vi "stop.vi"(8 "error in (no error)":errorcluster, 10 "stop?":bool, 11 "BECHWCBasic in":refnum<class "BECHWCBasic.lvclass">) -> (0 "error out":errorcluster, 2 "stopped":bool, 3 "BECHWCBasic out":refnum<class "BECHWCBasic.lvclass">)   [LabVIEW 2011, in "Hardware.lvlib" / "HWControllers.lvlib" / "BECHWCBasic.lvclass"]
doc: "Stop current run if input is true, otherwise ask hardware if its finished."
uses:
  BECHWCBasic.lvclass
  BECHWCBasic.lvclass/BECHWCBasic.ctl
  Channels/Digital/DigitalOutput.lvclass
  Channels/VoltOutput/AnalogOutput.lvclass
  IntegrationManagement/CameraManager.lvclass
  HWController.lvclass
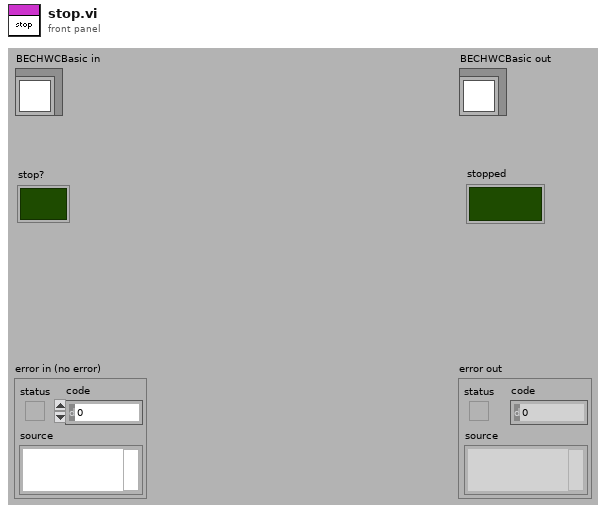
[diagram p1: front panel]
types:
  T1 = enum16{"Ready", "Compiling", "Configured", "Running", "Stopping", "Unresolved Error"}
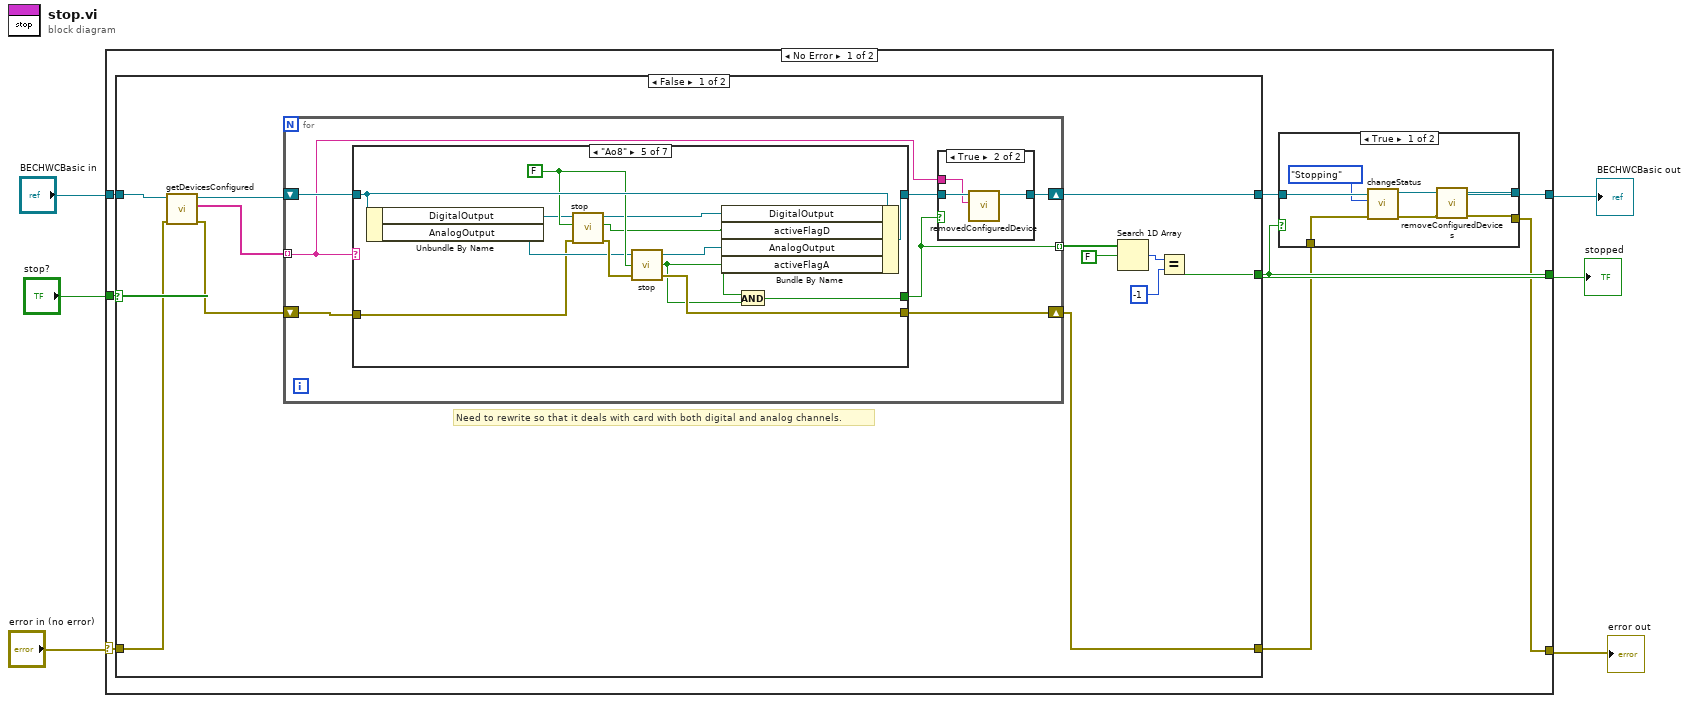
[diagram p0: block diagram]
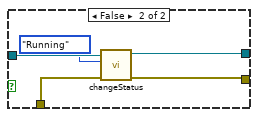
[diagram p2: hidden frame]
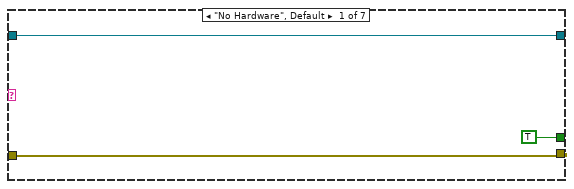
[diagram p4: hidden frame]
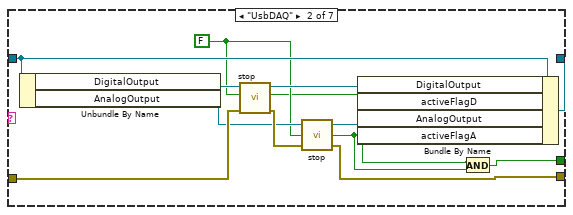
[diagram p5: hidden frame]
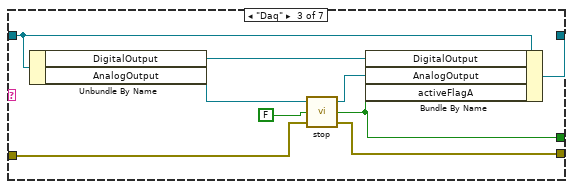
[diagram p6: hidden frame]
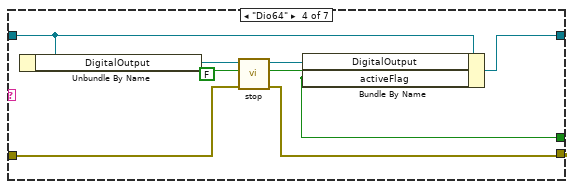
[diagram p7: hidden frame]
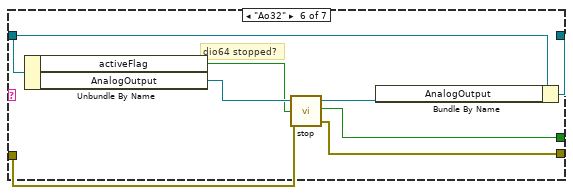
[diagram p8: hidden frame]
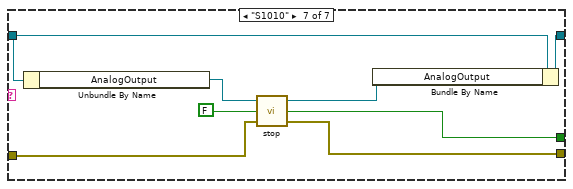
[diagram p9: hidden frame]
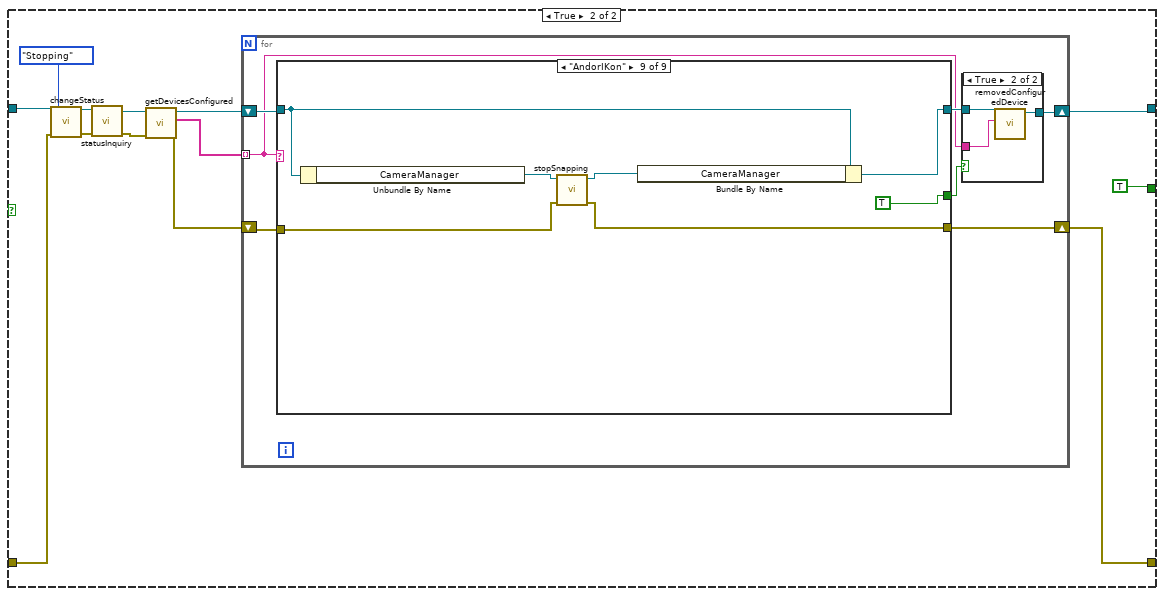
[diagram p10: hidden frame]
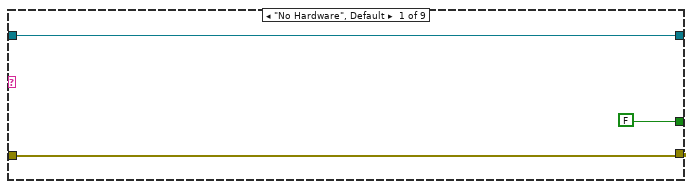
[diagram p12: hidden frame]
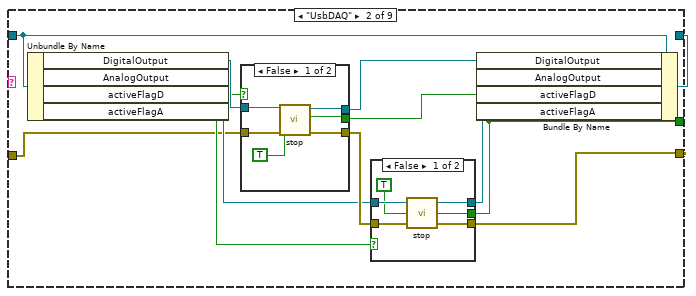
[diagram p13: hidden frame]
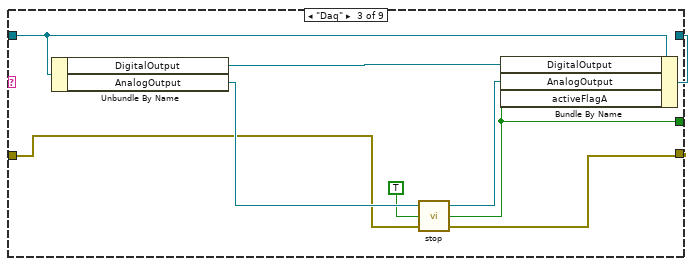
[diagram p16: hidden frame]
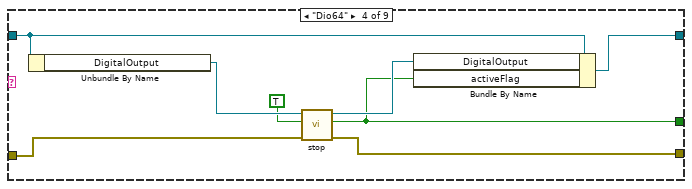
[diagram p17: hidden frame]
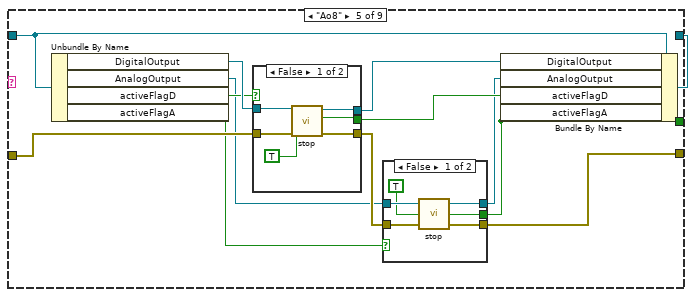
[diagram p18: hidden frame]
diagram:
  n1 = case shown="No Error" "error in (no error)" {
    selector: "error in (no error)" -> [w13 w247]
    tunnel: "BECHWCBasic in" -> [w14 w248]
    tunnel: [w8 w248] -> w5
    tunnel: [w7 w247] -> w3
    tunnel: "stop?" -> [w12 _]
    tunnel: [w9 _] -> w1
    frame No Error {
      n2 = case shown="False" w12 {
        tunnel: w14 -> [w31 w124]
        tunnel: [w38 w122] -> w11
        tunnel: w13 -> [w29 w123]
        tunnel: [w37 w121] -> w10
        tunnel: [w32 TRUE] -> w9
        frame False {
          # "Need to rewrite so that it deals with card with both digital and analog channels."
          n3 = call "getDevicesConfigured.vi"("error in (no error)"=w29, "HWController.lvclass in"=w31) -> ("error out"=w28:errorcluster, "devicesConfigured"=w27:string[], "HWController.lvclass out"=w30:refnum<class "BECHWCBasic.lvclass">)  [unwired: 7 in]
          n4 = for {
            shift-right: [w40] -> w38
            shift-left: w30 -> [w45]
            tunnel: w27 -> [w41] mode=indexing
            shift-right: [w44] -> w37
            shift-left: w28 -> [w43]
            tunnel: [w42] -> w36 mode=indexing
            n5 = case shown="\"Ao8\"" w41 {
              tunnel: [w52 w64 w74 w78 w94 w103 w111] -> w39
              tunnel: [w51 w61 w69 w80 w87 w100 w108] -> w44
              tunnel: w45 -> [w52 w65 w72 w77 w95 w102 w110]
              tunnel: w43 -> [w51 w59 w66 w81 w88 w98 w106]
              tunnel: [TRUE w53 w67 w75 w83 w97 w104] -> w42
              frame "No Hardware", Default {
              }
              frame "UsbDAQ" {
                w57 = FALSE
                n6 = Unbundle By Name(w65) -> ("DigitalOutput"=w63:refnum<class "DigitalOutput.lvclass">, "AnalogOutput"=w58:refnum<class "AnalogOutput.lvclass">)
                n7 = call-dynamic "stop.vi"("error in (no error)"=w59, "stop"=w57, "DigitalOutput in"=w63) -> ("error out"=w60:errorcluster, "stopped"=w54:bool, "DigitalOutput out"=w62:refnum<class "DigitalOutput.lvclass">)  [unwired: 6 in]
                n8 = call-dynamic "stop.vi"("error in (no error)"=w60, "stop"=w57, "AnalogOutput in"=w58) -> ("error out"=w61:errorcluster, "Stopped"=w55:bool, "AnalogOutput out"=w56:refnum<class "AnalogOutput.lvclass">)
                n9 = Bundle By Name(cluster=w65, "DigitalOutput"=w62, "activeFlagD"=w54, "AnalogOutput"=w56, "activeFlagA"=w55) -> (w64:refnum<class "BECHWCBasic.lvclass">)
                n10 = And(x=w54, y=w55) -> (x .and. y?=w53:bool)
              }
              frame "Daq" {
                n11 = Unbundle By Name(w72) -> ("DigitalOutput"=w68:refnum<class "DigitalOutput.lvclass">, "AnalogOutput"=w71:refnum<class "AnalogOutput.lvclass">)
                n12 = call-dynamic "stop.vi"("error in (no error)"=w66, "stop"=FALSE, "AnalogOutput in"=w71) -> ("error out"=w69:errorcluster, "Stopped"=w67:bool, "AnalogOutput out"=w70:refnum<class "AnalogOutput.lvclass">)
                n13 = Bundle By Name(cluster=w72, "DigitalOutput"=w68, "AnalogOutput"=w70, "activeFlagA"=w67) -> (w74:refnum<class "BECHWCBasic.lvclass">)
              }
              frame "Dio64" {
                n14 = Unbundle By Name(w77) -> ("DigitalOutput"=w82:refnum<class "DigitalOutput.lvclass">)
                n15 = call-dynamic "stop.vi"("error in (no error)"=w81, "stop"=FALSE, "DigitalOutput in"=w82) -> ("error out"=w80:errorcluster, "stopped"=w75:bool, "DigitalOutput out"=w79:refnum<class "DigitalOutput.lvclass">)  [unwired: 6 in]
                n16 = Bundle By Name(cluster=w77, "DigitalOutput"=w79, "activeFlag"=w75) -> (w78:refnum<class "BECHWCBasic.lvclass">)
              }
              frame "Ao8" {
                w92 = FALSE
                n17 = Unbundle By Name(w95) -> ("DigitalOutput"=w91:refnum<class "DigitalOutput.lvclass">, "AnalogOutput"=w90:refnum<class "AnalogOutput.lvclass">)
                n18 = call-dynamic "stop.vi"("error in (no error)"=w88, "stop"=w92, "DigitalOutput in"=w91) -> ("error out"=w93:errorcluster, "stopped"=w85:bool, "DigitalOutput out"=w89:refnum<class "DigitalOutput.lvclass">)  [unwired: 6 in]
                n19 = call-dynamic "stop.vi"("error in (no error)"=w93, "stop"=w92, "AnalogOutput in"=w90) -> ("error out"=w87:errorcluster, "Stopped"=w84:bool, "AnalogOutput out"=w86:refnum<class "AnalogOutput.lvclass">)
                n20 = Bundle By Name(cluster=w95, "DigitalOutput"=w89, "activeFlagD"=w85, "AnalogOutput"=w86, "activeFlagA"=w84) -> (w94:refnum<class "BECHWCBasic.lvclass">)
                n21 = And(x=w85, y=w84) -> (x .and. y?=w83:bool)
              }
              frame "Ao32" {
                # "dio64 stopped?"
                n22 = Unbundle By Name(w102) -> ("activeFlag"=w96:bool, "AnalogOutput"=w101:refnum<class "AnalogOutput.lvclass">)
                n23 = call-dynamic "stop.vi"("error in (no error)"=w98, "stop"=w96, "AnalogOutput in"=w101) -> ("error out"=w100:errorcluster, "Stopped"=w97:bool, "AnalogOutput out"=w99:refnum<class "AnalogOutput.lvclass">)
                n24 = Bundle By Name(cluster=w102, "AnalogOutput"=w99) -> (w103:refnum<class "BECHWCBasic.lvclass">)
              }
              frame "S1010" {
                n25 = Unbundle By Name(w110) -> ("AnalogOutput"=w109:refnum<class "AnalogOutput.lvclass">)
                n26 = call-dynamic "stop.vi"("error in (no error)"=w106, "stop"=FALSE, "AnalogOutput in"=w109) -> ("error out"=w108:errorcluster, "Stopped"=w104:bool, "AnalogOutput out"=w107:refnum<class "AnalogOutput.lvclass">)
                n27 = Bundle By Name(cluster=w110, "AnalogOutput"=w107) -> (w111:refnum<class "BECHWCBasic.lvclass">)
              }
            }
            n28 = case shown="True" w42 {
              tunnel: w41 -> [_ w47]
              tunnel: [w46 w48] -> w40
              tunnel: w39 -> [w46 w49]
              frame False {
              }
              frame True {
                n29 = call-dynamic "removedConfiguredDevice.vi"("device"=w47, "HWController in"=w49) -> ("HWController out"=w48:refnum<class "BECHWCBasic.lvclass">)  [unwired: 8 in, 1 out]
              }
            }
          }
          n30 = Search 1D Array(1D array=w36, element=FALSE) -> (index of element=w34:i32)  [unwired: 1 in]
          n31 = Equal?(x=w34, y=-1) -> (x = y?=w32:bool)
        }
        frame True {
          n32 = call "changeStatus.vi"("error in (no error)"=w123, "status"=T1."Stopping", "HWController in"=w124) -> ("error out"=w118:errorcluster, "HWController out"=w119:refnum<class "BECHWCBasic.lvclass">)  [unwired: 7 in]
          n33 = call-dynamic "statusInquiry.vi"("error in (no error)"=w118, "HWController in"=w119) -> ("error out"=w114:errorcluster, "HWController out"=w117:refnum<class "BECHWCBasic.lvclass">)  [unwired: 8 in]
          n34 = call "getDevicesConfigured.vi"("error in (no error)"=w114, "HWController.lvclass in"=w117) -> ("error out"=w113:errorcluster, "devicesConfigured"=w115:string[], "HWController.lvclass out"=w116:refnum<class "BECHWCBasic.lvclass">)  [unwired: 7 in]
          n35 = for {
            tunnel: w115 -> [w126] mode=indexing
            shift-right: [w127] -> w122
            shift-left: w116 -> [w131]
            shift-right: [w129] -> w121
            shift-left: w113 -> [w130]
            n36 = case shown="\"AndorIKon\"" w126 {
              tunnel: [w138 w143 w176 w181 w199 w224 w227 w234 w241] -> w128
              tunnel: [w137 w140 w174 w184 w190 w221 w230 w235 w242] -> w129
              tunnel: w131 -> [w138 w142 w175 w182 w198 w223 w228 w237 w244]
              tunnel: w130 -> [w137 w141 w171 w185 w196 _ w231 w238 w245]
              tunnel: [FALSE w139 w173 w180 w188 w218 w226 TRUE TRUE] -> w125
              frame "No Hardware", Default {
              }
              frame "UsbDAQ" {
                n37 = Unbundle By Name(w142) -> ("DigitalOutput"=w151:refnum<class "DigitalOutput.lvclass">, "AnalogOutput"=w147:refnum<class "AnalogOutput.lvclass">, "activeFlagD"=w150:bool, "activeFlagA"=w146:bool)
                n38 = case shown="False" w150 {
                  selector: w150 -> [_ w167]
                  tunnel: w151 -> [w166 w169]
                  tunnel: [w165 w169] -> w149
                  tunnel: w141 -> [w164 w168]
                  tunnel: [w163 w168] -> w148
                  tunnel: [w161 w167] -> w145
                  frame False {
                    n39 = call-dynamic "stop.vi"("error in (no error)"=w164, "stop"=TRUE, "DigitalOutput in"=w166) -> ("error out"=w163:errorcluster, "stopped"=w161:bool, "DigitalOutput out"=w165:refnum<class "DigitalOutput.lvclass">)  [unwired: 6 in]
                  }
                  frame True {
                  }
                }
                n40 = case shown="False" w146 {
                  selector: w146 -> [_ w158]
                  tunnel: w148 -> [w157 w159]
                  tunnel: w147 -> [w156 w160]
                  tunnel: [w154 w160] -> w144
                  tunnel: [w153 w159] -> w140
                  tunnel: [w152 w158] -> w139
                  frame False {
                    n41 = call-dynamic "stop.vi"("error in (no error)"=w157, "stop"=TRUE, "AnalogOutput in"=w156) -> ("error out"=w153:errorcluster, "Stopped"=w152:bool, "AnalogOutput out"=w154:refnum<class "AnalogOutput.lvclass">)
                  }
                  frame True {
                  }
                }
                n42 = Bundle By Name(cluster=w142, "DigitalOutput"=w149, "AnalogOutput"=w144, "activeFlagD"=w145, "activeFlagA"=w139) -> (w143:refnum<class "BECHWCBasic.lvclass">)
              }
              frame "Daq" {
                n43 = Unbundle By Name(w175) -> ("DigitalOutput"=w172:refnum<class "DigitalOutput.lvclass">, "AnalogOutput"=w178:refnum<class "AnalogOutput.lvclass">)
                n44 = call-dynamic "stop.vi"("error in (no error)"=w171, "stop"=TRUE, "AnalogOutput in"=w178) -> ("error out"=w174:errorcluster, "Stopped"=w173:bool, "AnalogOutput out"=w177:refnum<class "AnalogOutput.lvclass">)
                n45 = Bundle By Name(cluster=w175, "DigitalOutput"=w172, "AnalogOutput"=w177, "activeFlagA"=w173) -> (w176:refnum<class "BECHWCBasic.lvclass">)
              }
              frame "Dio64" {
                n46 = Unbundle By Name(w182) -> ("DigitalOutput"=w186:refnum<class "DigitalOutput.lvclass">)
                n47 = call-dynamic "stop.vi"("error in (no error)"=w185, "stop"=TRUE, "DigitalOutput in"=w186) -> ("error out"=w184:errorcluster, "stopped"=w180:bool, "DigitalOutput out"=w183:refnum<class "DigitalOutput.lvclass">)  [unwired: 6 in]
                n48 = Bundle By Name(cluster=w182, "DigitalOutput"=w183, "activeFlag"=w180) -> (w181:refnum<class "BECHWCBasic.lvclass">)
              }
              frame "Ao8" {
                n49 = Unbundle By Name(w198) -> ("DigitalOutput"=w197:refnum<class "DigitalOutput.lvclass">, "AnalogOutput"=w192:refnum<class "AnalogOutput.lvclass">, "activeFlagD"=w195:bool, "activeFlagA"=w187:bool)
                n50 = case shown="False" w195 {
                  selector: w195 -> [_ w215]
                  tunnel: w197 -> [w214 w217]
                  tunnel: [w213 w217] -> w194
                  tunnel: w196 -> [w212 w216]
                  tunnel: [w211 w216] -> w193
                  tunnel: [w209 w215] -> w191
                  frame False {
                    n51 = call-dynamic "stop.vi"("error in (no error)"=w212, "stop"=TRUE, "DigitalOutput in"=w214) -> ("error out"=w211:errorcluster, "stopped"=w209:bool, "DigitalOutput out"=w213:refnum<class "DigitalOutput.lvclass">)  [unwired: 6 in]
                  }
                  frame True {
                  }
                }
                n52 = case shown="False" w187 {
                  selector: w187 -> [_ w206]
                  tunnel: w193 -> [w205 w207]
                  tunnel: w192 -> [w204 w208]
                  tunnel: [w202 w208] -> w189
                  tunnel: [w201 w207] -> w190
                  tunnel: [w200 w206] -> w188
                  frame False {
                    n53 = call-dynamic "stop.vi"("error in (no error)"=w205, "stop"=TRUE, "AnalogOutput in"=w204) -> ("error out"=w201:errorcluster, "Stopped"=w200:bool, "AnalogOutput out"=w202:refnum<class "AnalogOutput.lvclass">)
                  }
                  frame True {
                  }
                }
                n54 = Bundle By Name(cluster=w198, "DigitalOutput"=w194, "AnalogOutput"=w189, "activeFlagD"=w191, "activeFlagA"=w188) -> (w199:refnum<class "BECHWCBasic.lvclass">)
              }
              frame "Ao32" {
                n55 = Unbundle By Name(w223) -> ("AnalogOutput"=w222:refnum<class "AnalogOutput.lvclass">)
                n56 = call-dynamic "stop.vi"("stop"=TRUE, "AnalogOutput in"=w222) -> ("error out"=w221:errorcluster, "Stopped"=w218:bool, "AnalogOutput out"=w220:refnum<class "AnalogOutput.lvclass">)  [unwired: 1 in]
                n57 = Bundle By Name(cluster=w223, "AnalogOutput"=w220) -> (w224:refnum<class "BECHWCBasic.lvclass">)
              }
              frame "S1010" {
                n58 = Unbundle By Name(w228) -> ("AnalogOutput"=w232:refnum<class "AnalogOutput.lvclass">)
                n59 = call-dynamic "stop.vi"("error in (no error)"=w231, "stop"=TRUE, "AnalogOutput in"=w232) -> ("error out"=w230:errorcluster, "Stopped"=w226:bool, "AnalogOutput out"=w229:refnum<class "AnalogOutput.lvclass">)
                n60 = Bundle By Name(cluster=w228, "AnalogOutput"=w229) -> (w227:refnum<class "BECHWCBasic.lvclass">)
              }
              frame "ICCamera" {
                n61 = Unbundle By Name(w237) -> ("CameraManager"=w239:refnum<class "CameraManager.lvclass">)
                n62 = call-dynamic "stopSnapping.vi"("error in (no error)"=w238, "CameraManager in"=w239) -> ("error out"=w235:errorcluster, "CameraManager out"=w236:refnum<class "CameraManager.lvclass">)  [unwired: 8 in]
                n63 = Bundle By Name(cluster=w237, "CameraManager"=w236) -> (w234:refnum<class "BECHWCBasic.lvclass">)
              }
              frame "AndorIKon" {
                n64 = Unbundle By Name(w244) -> ("CameraManager"=w246:refnum<class "CameraManager.lvclass">)
                n65 = call-dynamic "stopSnapping.vi"("error in (no error)"=w245, "CameraManager in"=w246) -> ("error out"=w242:errorcluster, "CameraManager out"=w243:refnum<class "CameraManager.lvclass">)  [unwired: 8 in]
                n66 = Bundle By Name(cluster=w244, "CameraManager"=w243) -> (w241:refnum<class "BECHWCBasic.lvclass">)
              }
            }
            n67 = case shown="True" w125 {
              tunnel: w128 -> [w132 w135]
              tunnel: [w132 w134] -> w127
              tunnel: w126 -> [_ w133]
              frame False {
              }
              frame True {
                n68 = call-dynamic "removedConfiguredDevice.vi"("device"=w133, "HWController in"=w135) -> ("HWController out"=w134:refnum<class "BECHWCBasic.lvclass">)  [unwired: 8 in, 1 out]
              }
            }
          }
        }
      }
      n69 = case shown="True" w9 {
        tunnel: w11 -> [w21 w26]
        tunnel: [w15 w25] -> w8
        tunnel: w10 -> [w20 w24]
        tunnel: [w16 w23] -> w7
        frame True {
          n70 = call "changeStatus.vi"("error in (no error)"=w20, "status"=T1."Stopping", "HWController in"=w21) -> ("error out"=w17:errorcluster, "HWController out"=w18:refnum<class "BECHWCBasic.lvclass">)  [unwired: 7 in]
          n71 = call "removeConfiguredDevices.vi"("error in (no error)"=w17, "HWController in"=w18) -> ("error out"=w16:errorcluster, "HWController out"=w15:refnum<class "BECHWCBasic.lvclass">)  [unwired: 8 in]
        }
        frame False {
          n72 = call "changeStatus.vi"("error in (no error)"=w24, "status"=T1."Running", "HWController in"=w26) -> ("error out"=w23:errorcluster, "HWController out"=w25:refnum<class "BECHWCBasic.lvclass">)  [unwired: 7 in]
        }
      }
    }
    frame Error {
    }
  }
  "error out" <- w3
  "BECHWCBasic out" <- w5
  "stopped" <- w1
